vi "Robot Moving.vi"(6 "Priority level array":dbl[][](array[numeric]), 8 "error in (no error)":errorcluster, 9 "location":dbl[](array[numeric]), 10 "direction":string) -> (0 "error out":errorcluster, 2 "new location":dbl[](array[numeric]), 3 "new direction":string)   [LabVIEW 2015]
uses:
  <vilib>/myRIO/Instrument Drivers/Onboard IO/PWM/typedefs/PWM Reference.ctl
  <vilib>/myRIO/Common/Instrument Driver Framework/Utilities/typedefs/myRIO Generic Hardware Reference.ctl
  <vilib>/myRIO/Common/Instrument Driver Framework/Utilities/typedefs/Hardware Version Enum.ctl
  <vilib>/myRIO/Common/Instrument Driver Framework/Utilities/typedefs/myRIO v1.0 Reference.ctl
  <vilib>/myRIO/Common/Instrument Driver Framework/Utilities/typedefs/Generic FPGA Reference.ctl
  <vilib>/myRIO/Common/Instrument Driver Framework/myRIO v1.0/PWM/typedefs/PWM Channels Enum.ctl
  <vilib>/myRIO/Instrument Drivers/Onboard IO/PWM/typedefs/PWM Configuration.ctl
  <vilib>/userdefined/High Color/nirio_resource_hc.ctl
  <vilib>/myRIO/Common/Instrument Driver Framework/Utilities/vis/Is FPGA Ref Available.vi
  <vilib>/myRIO/Common/Instrument Driver Framework/myRIO v1.0/PWM/vis/myRIO v1.1 Open PWM.vi
  <vilib>/myRIO/Instrument Drivers/Onboard IO/PWM/vis/Set Duty Cycle and Frequency.vi
  <vilib>/myRIO/Common/Instrument Driver Framework/Utilities/vis/Validate Channels.vi
  <vilib>/myRIO/Common/Instrument Driver Framework/myRIO v1.0/PWM/vis/myRIO v1.0 Reserve PWM.vi
  <vilib>/myRIO/Common/Instrument Driver Framework/myRIO v1.0/PWM/vis/myRIO v1.0 Build MUX Configuration PWM.vi
  <vilib>/myRIO/Common/Instrument Driver Framework/myRIO v1.0/Resource Manager/vis/myRIO v1.0 Reserve Channel List.vi
  <vilib>/myRIO/Common/Instrument Driver Framework/myRIO v1.0/Resource Manager/vis/myRIO v1.0 Create Configuration List.vi
  <vilib>/myRIO/Common/Instrument Driver Framework/myRIO v1.0/Resource Manager/vis/myRIO v1.0 Reserve Channel.vi
  <vilib>/myRIO/Common/Instrument Driver Framework/myRIO v1.0/Resource Manager/vis/myRIO v1.0 Unreserve Channel.vi
  <vilib>/myRIO/Common/Instrument Driver Framework/myRIO v1.0/Resource Manager/vis/myRIO v1.0 Build Mutex Name.vi
  <vilib>/Utility/VariantDataType/GetNumericInfo.vi
  <vilib>/Utility/error.llb/Error Cluster From Error Code.vi
  <vilib>/myRIO/Common/Instrument Driver Framework/myRIO v1.0/myRIO v1.1 Open.vi
  <vilib>/myRIO/Common/Instrument Driver Framework/Utilities/vis/IO Manager.vi
  <vilib>/myRIO/Common/Instrument Driver Framework/Utilities/vis/Configuration Manager.vi
  <vilib>/myRIO/Common/Instrument Driver Framework/myRIO v1.0/Resource Manager/vis/myRIO v1.0 Configure IO.vi
  <vilib>/myRIO/Common/Instrument Driver Framework/myRIO v1.0/myRIO v1.0 Close.vi
  <vilib>/myRIO/Common/Instrument Driver Framework/myRIO v1.0/PWM/vis/myRIO v1.0 Write PWM.vi
  <vilib>/myRIO/Express VI/Onboard IO/PWM/PWM Express VI.xnode
  <vilib>/myRIO/Instrument Drivers/Onboard IO/PWM/vis/myRIO PWM Open.xnode
  <vilib>/myRIO/Instrument Drivers/Onboard IO/PWM/PWM.lvlib
panel:
  out "error out 3":errorcluster
  out "error out 2":errorcluster
  in  "error in (no error) 3":errorcluster
  in  "error in (no error) 2":errorcluster
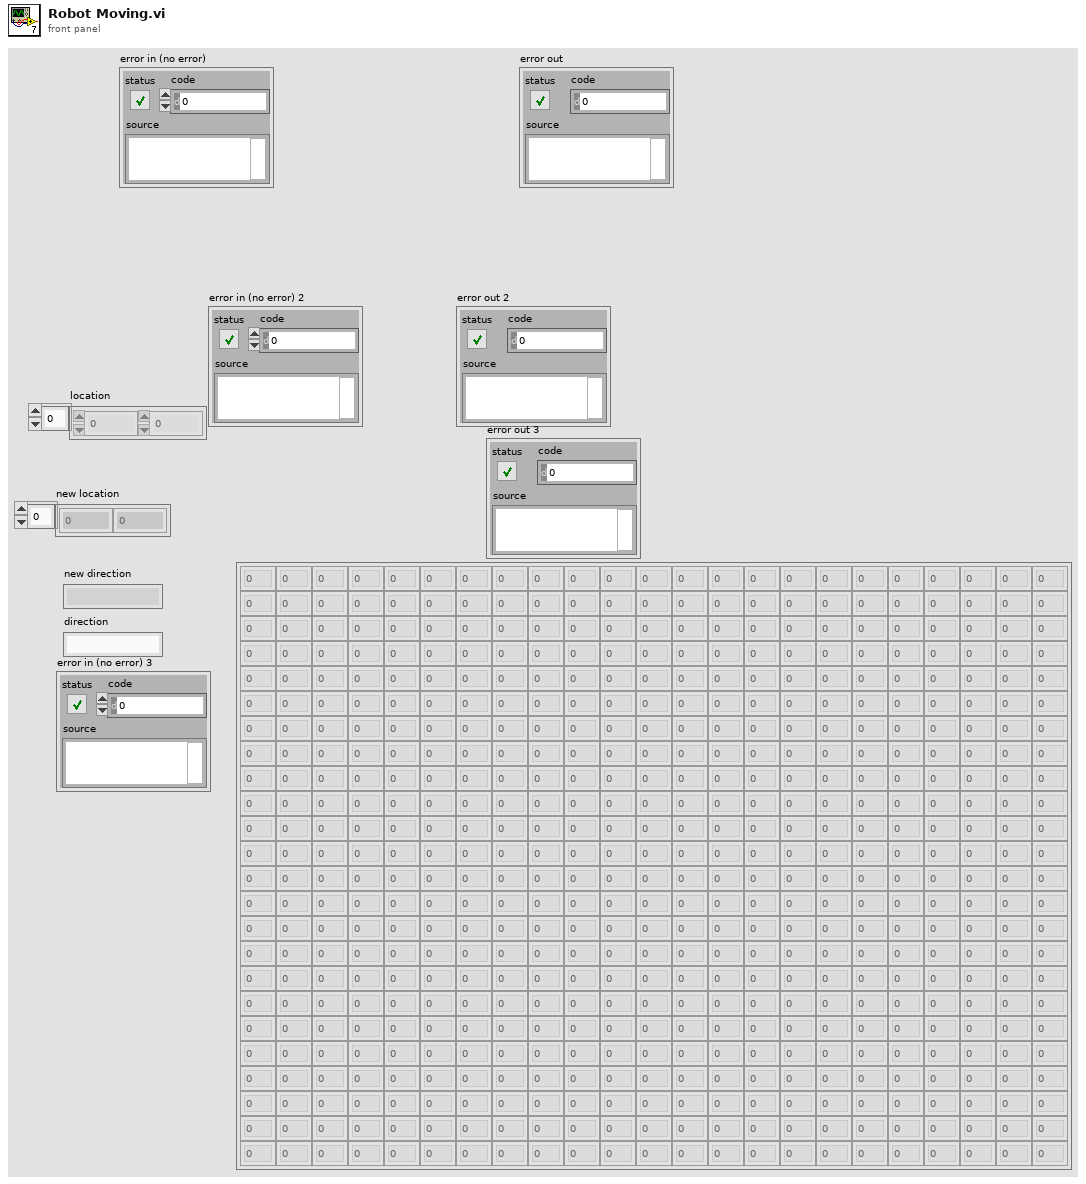
[diagram p1: front panel]
types:
  T1 = typedef "PWM.lvlib/PWM Reference.ctl" = cluster{"myRIO Reference":T2, "PWM Channels Enum":T6, "PWM Configuration":T7}
  T2 = typedef "myRIO Generic Hardware Reference.ctl" = cluster{"myRIO Model":T3, "myRIO Hardware Reference":T4}
  T3 = typedef "Hardware Version Enum.ctl" = enum16{"Unknown", "myRIO-1900", "myRIO-1950", "roboRIO"}
  T4 = typedef "myRIO v1.0 Reference.ctl" = cluster{"Generic FPGA Reference":T5, "Allow multiple opens":bool}
  T5 = typedef "Generic FPGA Reference.ctl" = refnum<k20>
  T6 = typedef "PWM Channels Enum.ctl" = enum16{"Not Connected", "C/PWM0", "C/PWM1", "A/PWM0", "A/PWM1", "A/PWM2", "B/PWM0", "B/PWM1", "B/PWM2", "PWM/PWM0", "PWM/PWM1", "PWM/PWM2", "PWM/PWM3", "PWM/PWM4", "PWM/PWM5", "PWM/PWM6", "PWM/PWM7", "PWM/PWM8", "PWM/PWM9"}
  T7 = typedef "PWM.lvlib/PWM Configuration.ctl" = cluster{"Frequency":dbl, "Duty Cycle":dbl}
  T8 = typedef "nirio_resource_hc.ctl" = tag
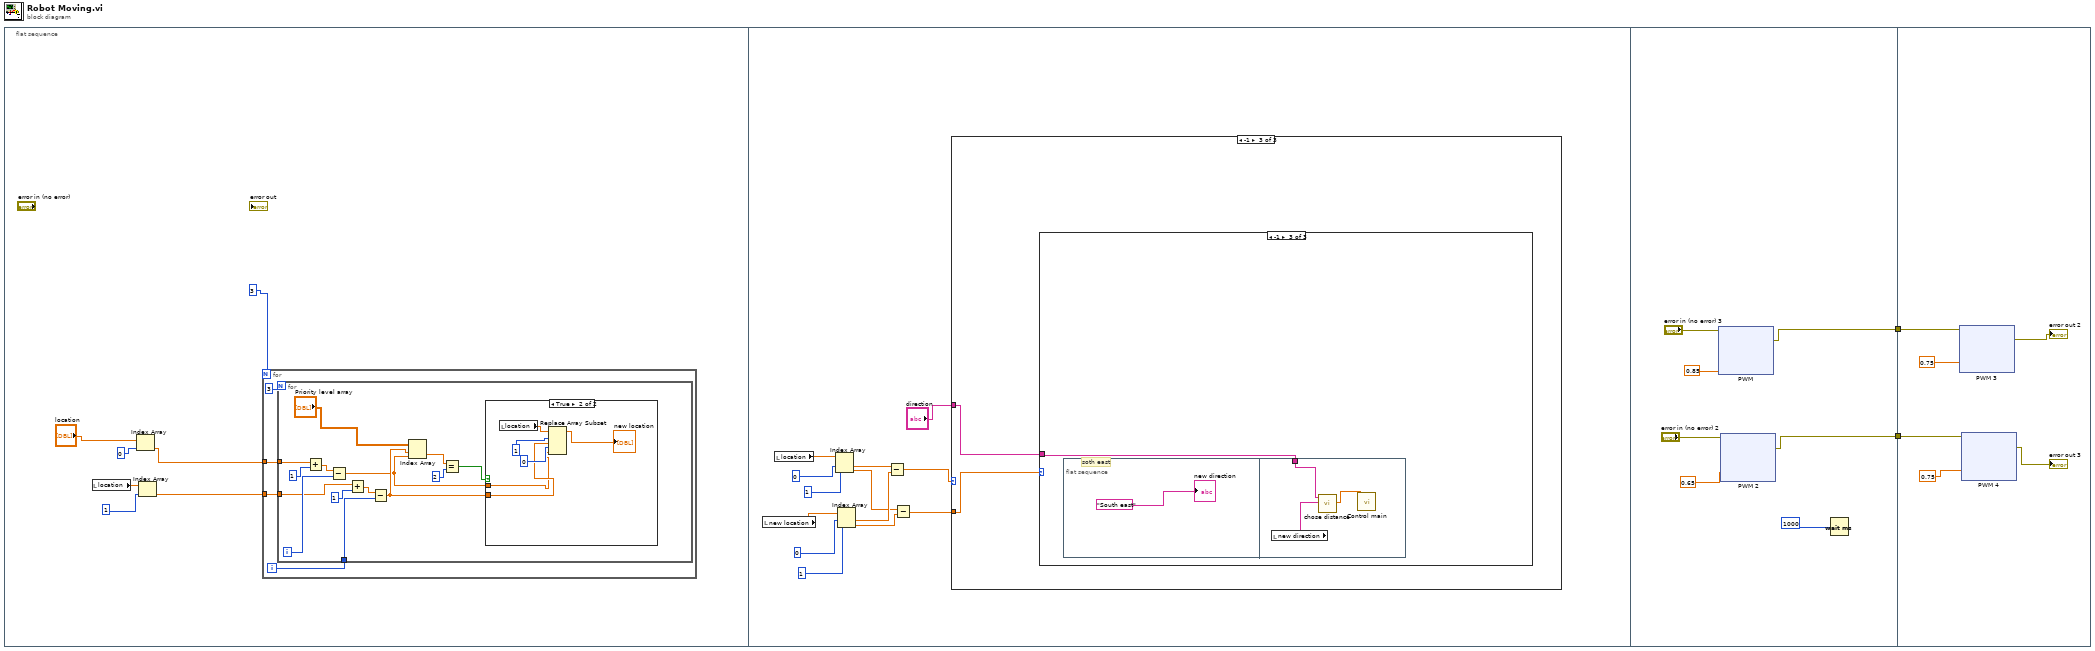
[diagram p0: block diagram]
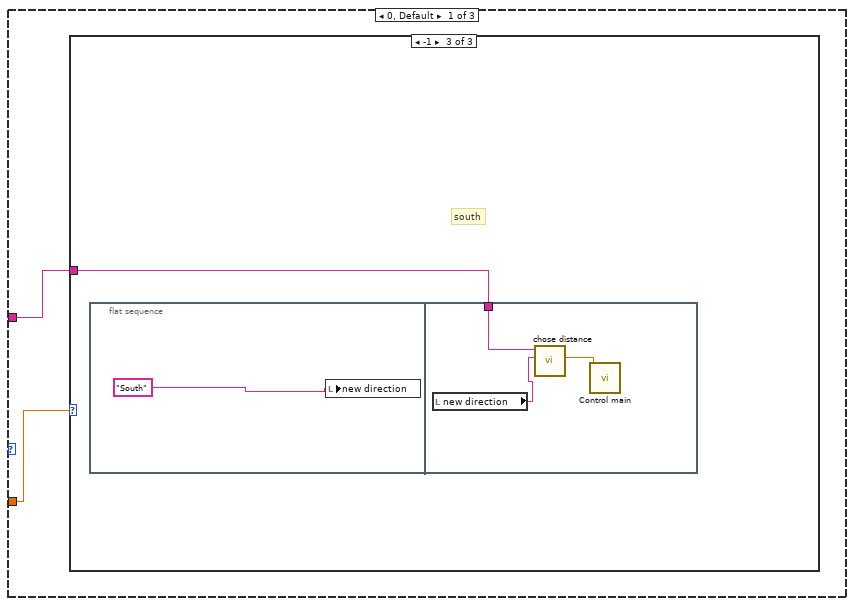
[diagram p3: hidden frame]
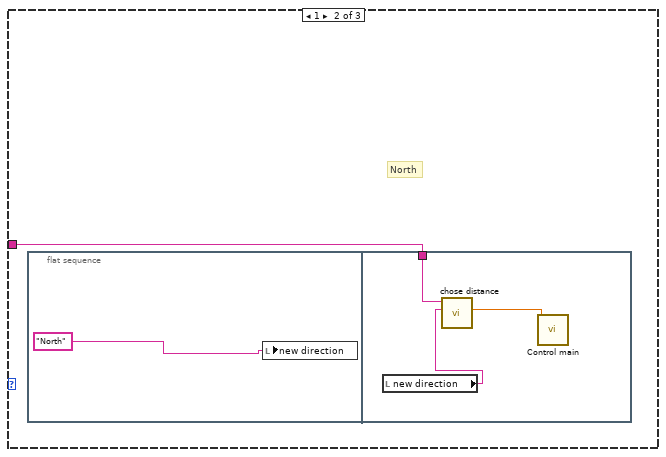
[diagram p5: hidden frame]
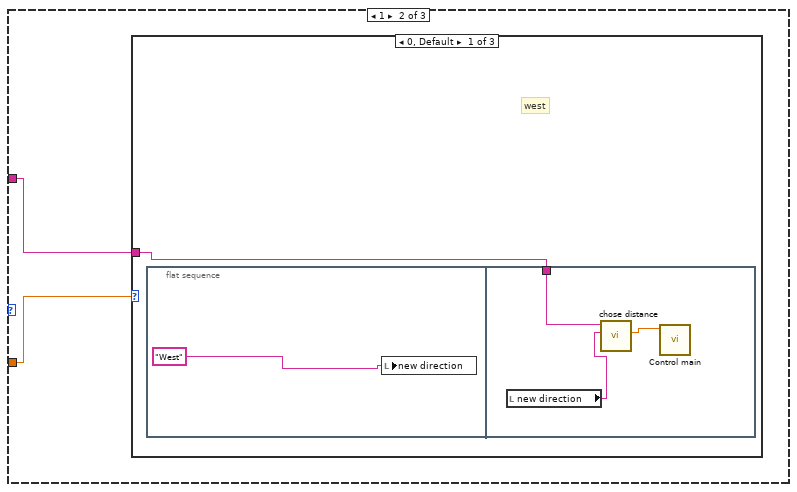
[diagram p6: hidden frame]
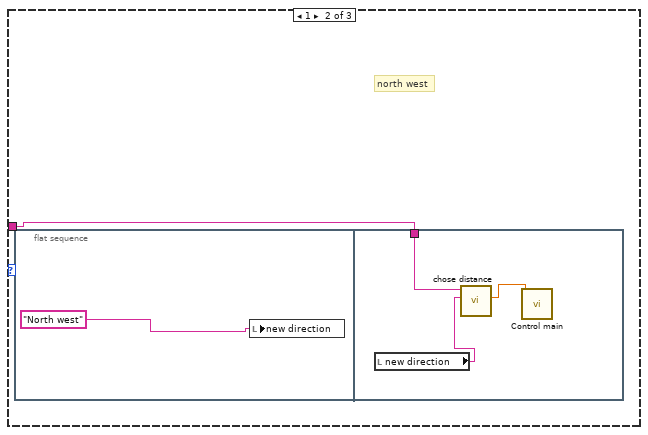
[diagram p7: hidden frame]
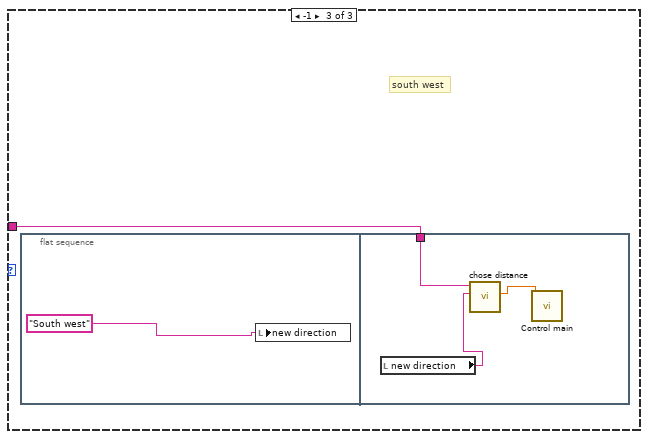
[diagram p8: hidden frame]
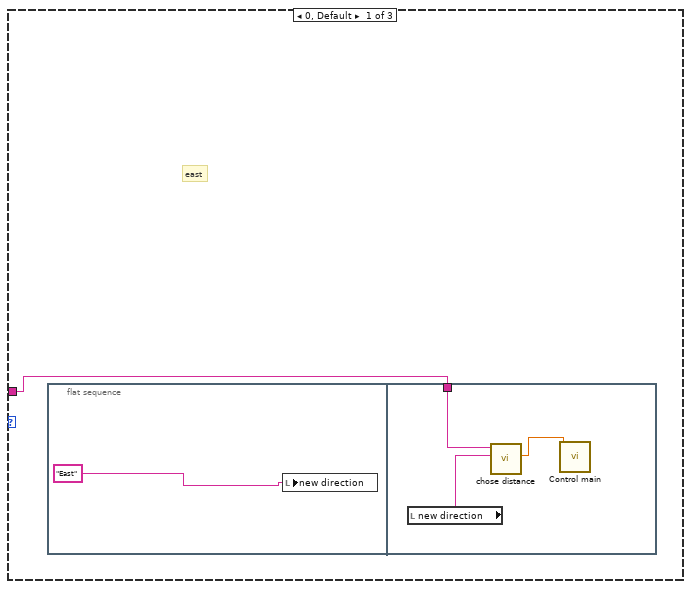
[diagram p9: hidden frame]
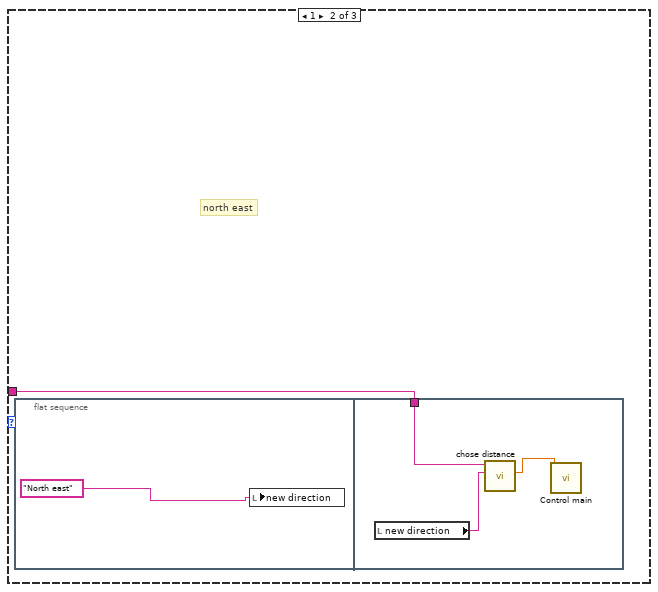
[diagram p10: hidden frame]
diagram:
  n1 = flat-sequence {
    tunnel: [w94] -> w2
    tunnel: [w93] -> w1
    tunnel: w2 -> [w175]
    tunnel: w1 -> [w174]
    frame #0 {
      n2 = local read "location"() -> (w8:dbl[])
      n3 = Index Array(array="location", index=0) -> (element=w5:dbl)
      n4 = Index Array(array=w8, index=1) -> (element=w4:dbl)
      n5 = for {
        N: 3 -> [_]
        tunnel: w5 -> [w11]
        tunnel: w4 -> [w10]
        i -> [w12]
        n6 = for {
          N: 3 -> [_]
          tunnel: w12 -> [w22]
          tunnel: w11 -> [w21]
          tunnel: w10 -> [w20]
          i -> [w25]
          n7 = Add(x=w21, y=1) -> (x+y=w26:dbl)
          n8 = Subtract(x=w26, y=w25) -> (x-y=w14:dbl)
          n9 = Add(x=w20, y=1) -> (x+y=w23:dbl)
          n10 = Subtract(x=w23, y=w22) -> (x-y=w16:dbl)
          n11 = Index Array(array="Priority level array", index (row)=w16, index (col)=w14) -> (element=w19:dbl)
          n12 = Equal?(x=w19, y=2) -> (x = y?=w17:bool)
          n13 = case shown="True" w17 {
            tunnel: w14 -> [_ w30]
            tunnel: w16 -> [_ w31]
            frame False {
            }
            frame True {
              n14 = local read "location"() -> (w29:dbl[])
              n15 = Replace Array Subset(array=w29, new element #1=w31, index #1=1, new element #2=w30, index #2=0) -> (→"new location":dbl[])
            }
          }
        }
      }
    }
    frame #1 {
      n16 = local read "new location"() -> (w43:dbl[])
      n17 = local read "location"() -> (w46:dbl[])
      n18 = Index Array(array=w46, index #1=0, index #2=1) -> (element #1=w40:dbl, element #2=w38:dbl)
      n19 = Index Array(array=w43, index #1=0, index #2=1) -> (element #1=w39:dbl, element #2=w37:dbl)
      n20 = Subtract(x=w40, y=w39) -> (x-y=w35:dbl)
      n21 = Subtract(x=w38, y=w37) -> (x-y=w36:dbl)
      n22 = case shown="-1" w35 {
        tunnel: w36 -> [w48 w60 w77]
        tunnel: "direction" -> [w47 w59 w76]
        frame 0, Default {
          n23 = case shown="-1" w48 {
            tunnel: w47 -> [_ w49 w54]
            frame 0, Default {
              # "Nothing"
            }
            frame 1 {
              # "North"
              n24 = flat-sequence {
                tunnel: w49 -> [w53]
                frame #0 {
                  n25 = local write "new direction"("North") -> ()
                }
                frame #1 {
                  n26 = local read "new direction"() -> (w52:string)
                  n27 = call "chose distance.vi"("New direction"=w52, "Current Direction"=w53) -> ("chosen  distance"=w51:dbl)  [unwired: 9 in]
                  n28 = call "Control main.vi"("chosen  distance"=w51) -> ()  [unwired: 11 in]
                }
              }
            }
            frame -1 {
              # "south"
              n29 = flat-sequence {
                tunnel: w54 -> [w57]
                frame #0 {
                  n30 = local write "new direction"("South") -> ()
                }
                frame #1 {
                  n31 = local read "new direction"() -> (w58:string)
                  n32 = call "chose distance.vi"("New direction"=w58, "Current Direction"=w57) -> ("chosen  distance"=w56:dbl)  [unwired: 9 in]
                  n33 = call "Control main.vi"("chosen  distance"=w56) -> ()  [unwired: 11 in]
                }
              }
            }
          }
        }
        frame 1 {
          n34 = case shown="0, Default" w60 {
            tunnel: w59 -> [w61 w66 w71]
            frame 0, Default {
              # "west"
              n35 = flat-sequence {
                tunnel: w61 -> [w64]
                frame #0 {
                  n36 = local write "new direction"("West") -> ()
                }
                frame #1 {
                  n37 = local read "new direction"() -> (w65:string)
                  n38 = call "chose distance.vi"("New direction"=w65, "Current Direction"=w64) -> ("chosen  distance"=w63:dbl)  [unwired: 9 in]
                  n39 = call "Control main.vi"("chosen  distance"=w63) -> ()  [unwired: 11 in]
                }
              }
            }
            frame 1 {
              # "north west"
              n40 = flat-sequence {
                tunnel: w66 -> [w70]
                frame #0 {
                  n41 = local write "new direction"("North west") -> ()
                }
                frame #1 {
                  n42 = local read "new direction"() -> (w69:string)
                  n43 = call "chose distance.vi"("New direction"=w69, "Current Direction"=w70) -> ("chosen  distance"=w68:dbl)  [unwired: 9 in]
                  n44 = call "Control main.vi"("chosen  distance"=w68) -> ()  [unwired: 11 in]
                }
              }
            }
            frame -1 {
              # "south west"
              n45 = flat-sequence {
                tunnel: w71 -> [w73]
                frame #0 {
                  n46 = local write "new direction"("South west") -> ()
                }
                frame #1 {
                  n47 = local read "new direction"() -> (w74:string)
                  n48 = call "chose distance.vi"("New direction"=w74, "Current Direction"=w73) -> ("chosen  distance"=w75:dbl)  [unwired: 9 in]
                  n49 = call "Control main.vi"("chosen  distance"=w75) -> ()  [unwired: 11 in]
                }
              }
            }
          }
        }
        frame -1 {
          n50 = case shown="-1" w77 {
            tunnel: w76 -> [w78 w83 w88]
            frame 0, Default {
              # "east"
              n51 = flat-sequence {
                tunnel: w78 -> [w82]
                frame #0 {
                  n52 = local write "new direction"("East") -> ()
                }
                frame #1 {
                  n53 = local read "new direction"() -> (w81:string)
                  n54 = call "chose distance.vi"("New direction"=w81, "Current Direction"=w82) -> ("chosen  distance"=w80:dbl)  [unwired: 9 in]
                  n55 = call "Control main.vi"("chosen  distance"=w80) -> ()  [unwired: 11 in]
                }
              }
            }
            frame 1 {
              # "north east"
              n56 = flat-sequence {
                tunnel: w83 -> [w86]
                frame #0 {
                  n57 = local write "new direction"("North east") -> ()
                }
                frame #1 {
                  n58 = local read "new direction"() -> (w87:string)
                  n59 = call "chose distance.vi"("New direction"=w87, "Current Direction"=w86) -> ("chosen  distance"=w85:dbl)  [unwired: 9 in]
                  n60 = call "Control main.vi"("chosen  distance"=w85) -> ()  [unwired: 11 in]
                }
              }
            }
            frame -1 {
              # "soth east"
              n61 = flat-sequence {
                tunnel: w88 -> [w91]
                frame #0 {
                  "new direction" <- "South east"
                }
                frame #1 {
                  n62 = local read "new direction"() -> (w92:string)
                  n63 = call "chose distance.vi"("New direction"=w92, "Current Direction"=w91) -> ("chosen  distance"=w90:dbl)  [unwired: 9 in]
                  n64 = call "Control main.vi"("chosen  distance"=w90) -> ()  [unwired: 11 in]
                }
              }
            }
          }
        }
      }
    }
    frame #2 {
      n65 = xnode "PWM"("Duty Cycle"=0.85, "error in (no error)"="error in (no error) 3") -> ("error out"=w94:errorcluster)
      n66 = xnode "PWM 2"("Duty Cycle"=0.65 ("Duty Cycle 2"), "error in (no error)"="error in (no error) 2") -> ("error out"=w93:errorcluster)
      n67 = Wait (ms)(milliseconds to wait=1000) -> ()  [unwired: 1 out]
    }
    frame #3 {
      n68 = xnode "PWM 3"("Duty Cycle"=0.75, "error in (no error)"=w175) -> ("error out"=→"error out 2":errorcluster)
      n69 = xnode "PWM 4"("Duty Cycle"=0.75, "error in (no error)"=w174) -> ("error out"=→"error out 3":errorcluster)
    }
  }
